vi "Voltage Update.vi"(0 "Voltage Output (to Backgate)":dbl) -> ()   [LabVIEW 2013]
doc: "I. Description:\nThis example demonstrates how to output a single Voltage Update (Sample) to an Analog Output Channel.\n\nII. Instructions for Running:\n1. Select the Physical Channel to correspond to where your signal is output on the DAQ device.\n2. Enter the Minimum and Maximum Voltage Ranges\nNote: Use the Acq One Sample example to verify you are generating the correct output on the DAQ device\n\nIII. Block Diagram Steps:\n1. Create an Analog Output Voltage Channel\n2. Use the Write VI to Output 1 Sample to 1 Channel on the Data\nAcquisition Card. \n3. Call the Clear Task VI to clear the Task.\n4. Use the popup dialog box to display an error if any. \n\nIV. I/O Connections Overview:\nMake sure your signal output terminal matches the Physical Channel I/O Control. For further connection information, refer to your hardware reference manual."
uses:
  <vilib>/Utility/error.llb/DialogType.ctl
  Lock-in Globals Multiple Inputs and Outputs.vi
  <vilib>/DAQmx/create/channels.llb/DAQmx Create Channel (AO-Voltage-Basic).vi
  <vilib>/DAQmx/write.llb/DAQmx Write (Analog DBL 1Chan 1Samp).vi
panel:
  out "Gain":dbl=19.427 format="%0.2f"
  in  "Maximum Value":dbl=80.0 format="%0.2f"
  in  "Minimum Value":dbl=-80.0 format="%0.2f"
  in  "Physical Channel":tag="PXI1Slot2/ao0"
  # "Update Voltage for Backgate"
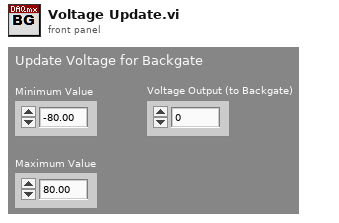
[diagram p1: front panel]
types:
  T1 = typedef "DialogType.ctl" = u16
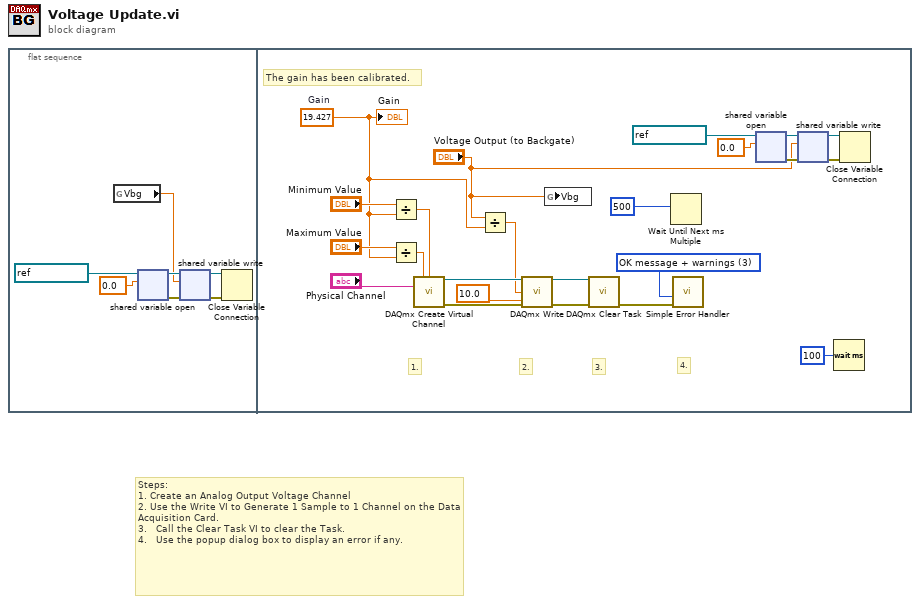
[diagram p0: block diagram]
diagram:
  # "Steps: \n1. Create an Analog Output Voltage Channel\n2. Use the Write VI to Generate 1 Sample to 1 Channel on the Data Acquisition Card.  \n3.   Call the Clear Task VI to clear the Task.\n4.   Use the popup dialog box to display an error if any."
  n1 = flat-sequence {
    frame #0 {
      n2 = global read "Lock-in Globals Multiple Inputs and Outputs.vi" "Vbg"() -> (w1:dbl)
      n3 = shared-variable-open(refnum<k21> "ni.var.psp://housesoftheholy/PPMS 2/PPMS 2 Vbg" ("shared variable refnum in"), 0.0 ("Gain")) -> (w7:refnum<k21>, w6:errorcluster)  [unwired: 2 in]
      n4 = shared-variable-write(w7, w6, w1) -> (w2:refnum<k21>, w3:errorcluster)
      n5 = Close Variable Connection(8:w3, 11:w2) -> ()  [unwired: 1 out]
    }
    frame #1 {
      w17 = 19.427  # Gain
      w26 = T1 3 items=["no dialog", "OK message", "continue or stop message", "OK message + warnings", "continue/stop + warnings"] ("type of dialog (OK msg:1)")
      # "The gain has been calibrated."
      # "4."
      # "2."
      # "3."
      # "1."
      n6 = Divide(x="Minimum Value", y=w17) -> (x/y=w20:dbl)
      n7 = Divide(x="Maximum Value", y=w17) -> (x/y=w18:dbl)
      n8 = call-poly <vilib>:"DAQmx Create Virtual Channel.vi"("maximum value"=w18, "minimum value"=w20, "physical channels"="Physical Channel") -> ("task out"=w28:refnum<k21>, "error out"=w29:errorcluster)  [unwired: 11 in]
      n9 = Divide(x="Voltage Output (to Backgate)", y=w17) -> (x/y=w16:dbl)
      n10 = call-poly <vilib>:"DAQmx Write.vi"("task/channels in"=w28, "data"=w16, "timeout"=10.0, "error in"=w29) -> ("task out"=w24:refnum<k21>, "error out"=w25:errorcluster)  [unwired: 9 in, 1 out]
      n11 = global write "Lock-in Globals Multiple Inputs and Outputs.vi" "Vbg"("Voltage Output (to Backgate)") -> ()
      n12 = call <vilib>:"DAQmx Clear Task.vi"("task in"=w24, "error in"=w25) -> ("error out"=w23:errorcluster)  [unwired: 13 in]
      n13 = Wait Until Next ms Multiple(millisecond multiple=u32 500 ("milliseconds to wait")) -> ()  [unwired: 1 out]
      n14 = call <vilib>:"Simple Error Handler.vi"("type of dialog (OK msg:1)"=w26, "error in (no error)"=w23) -> ()  [unwired: 3 in, 5 out]
      n15 = shared-variable-open(refnum<k21> "ni.var.psp://housesoftheholy/PPMS 2/PPMS 2 Vbg" ("shared variable refnum in"), 0.0 ("Gain")) -> (w15:refnum<k21>, w14:errorcluster)  [unwired: 2 in]
      n16 = shared-variable-write(w15, w14, "Voltage Output (to Backgate)") -> (w10:refnum<k21>, w11:errorcluster)
      n17 = Wait (ms)(milliseconds to wait=u32 100) -> ()  [unwired: 1 out]
      n18 = Close Variable Connection(8:w11, 11:w10) -> ()  [unwired: 1 out]
      "Gain" <- w17
    }
  }
